vi "GetCXT.vi"(7 "key description":string, 8 "sections":string[](array[string]), 9 "numeric":cxt=nan+nani, 11 "info data":string) -> (0 "sections out":string[](array[string]), 1 "key found?":bool, 2 "value":cxt format="%#_20g", 3 "info data out":string)   [LabVIEW 2020, in "infolib.lvlib"]
doc: "Add a new numeric key to Info Data string. If section exists in Info Data string, inserts key into this section."
uses:
  infolib.lvlib
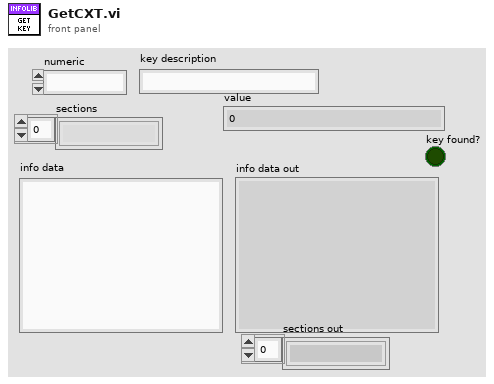
[diagram p1: front panel]
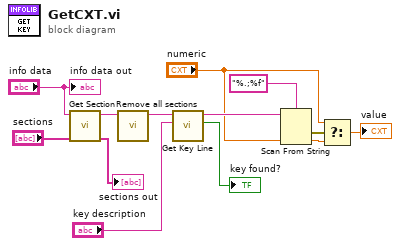
[diagram p0: block diagram]
diagram:
  n1 = call "Get Section.vi"("sections"="sections", "info data"="info data") -> ("sections out"=→"sections out":string[], "section part"=w13:string)  [unwired: 7 in, 1 out]
  n2 = call "Remove all sections.vi"("info data"=w13) -> ("info data out"=w12:string)  [unwired: 10 in]
  n3 = call "Get Key Line.vi"("key description"="key description", "info data"=w12) -> ("key found?"=→"key found?":bool, "key value"=w3:string)  [unwired: 8 in]
  n4 = Scan From String(format string="%.;%f", input string=w3, default 1="numeric") -> (error out=w5:errorcluster, output 1=w4:cxt)  [unwired: 2 in, 2 out]
  n5 = Select(t="numeric", s=w5, f=w4) -> (s? t:f=→"value":cxt)
  "info data out" <- "info data"
